vi "Update.vi"(8 "error in (no error)":errorcluster, 10 "Message in":refnum<class "UpdateMessage.lvclass">, 11 "StageSPIM in":refnum<class "StageSPIM.lvclass">) -> (0 "error out":errorcluster, 3 "StageSPIM out":refnum<class "StageSPIM.lvclass">)   [LabVIEW 2012, in "StageSPIM.lvclass"]
doc: "The update method processes the command 'update'. \n\nThe command 'update' is used for receiving new values to be set to the private data of the class. This could be seen as a public set method for setting new parameters to the private class data."
uses:
  StageSPIM.lvclass
  <vilib>/Distrio/Murmex/Murmex/Murmex.lvclass
  <vilib>/Distrio/Murmex/UpdateMessage/UpdateMessage.lvclass
panel:
  # "This method is called when the UPDATE\ntrigger is sent. \n\nOverride this method when your component needs to\nrespond to this trigger. \n\nCall parent for proper implementation"
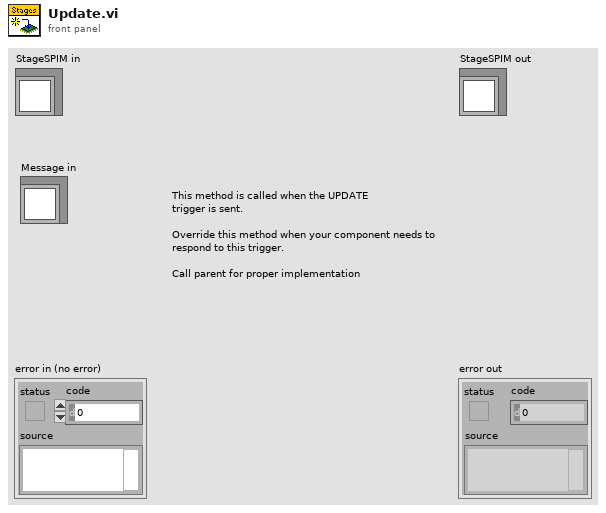
[diagram p1: front panel]
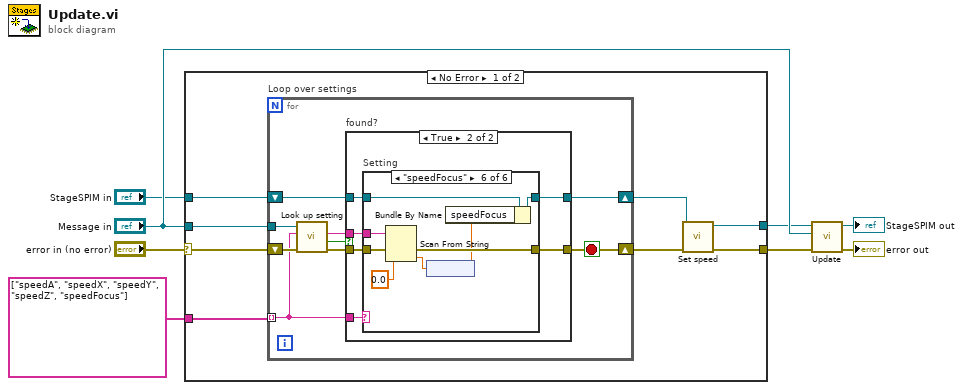
[diagram p0: block diagram]
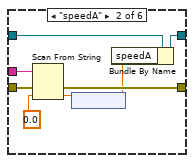
[diagram p4: hidden frame]
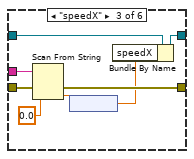
[diagram p5: hidden frame]
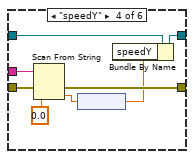
[diagram p6: hidden frame]
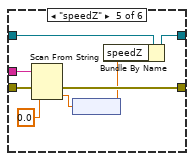
[diagram p7: hidden frame]
diagram:
  n1 = case shown="No Error" "error in (no error)" {
    selector: "error in (no error)" -> [w16 w76]
    tunnel: [w11 w76] -> w5
    tunnel: string[] ["speedA", "speedX", "speedY", "speedZ", "speedFocus"] ("key chains") -> [w15 _]
    tunnel: "Message in" -> [w14 _]
    tunnel: "StageSPIM in" -> [w13 w77]
    tunnel: [w9 w77] -> w1
    frame No Error {
      n2 = for "Loop over settings" {
        shift-right: [w17] -> w12
        shift-left: w16 -> [w25]
        tunnel: w15 -> [w19] mode=indexing
        tunnel: w14 -> [w24]
        shift-right: [w18] -> w10
        shift-left: w13 -> [w22]
        stop <- w17 stop-if-true
        n3 = call <vilib>:"Look up setting.vi"("error in (no error)"=w25, "tag name"=w19, "UpdateMessage in"=w24) -> ("error out"=w20:errorcluster, "found?"=w23:bool, "value"=w21:string)  [unwired: 5 in, 1 out]
        n4 = case "found?" shown="True" w23 {
          tunnel: w22 -> [w27 w31]
          tunnel: w21 -> [_ w32]
          tunnel: w20 -> [w26 w30]
          tunnel: w19 -> [_ w33]
          tunnel: [w27 w29] -> w18
          tunnel: [w26 w28] -> w17
          frame False {
          }
          frame True {
            n5 = case "Setting" shown="\"speedFocus\"" w33 {
              tunnel: w32 -> [_ w39 w50 w54 w63 w71]
              tunnel: w31 -> [w35 w41 w49 w58 w66 w74]
              tunnel: w30 -> [w34 w43 w51 w59 w67 w75]
              tunnel: [w35 w40 w48 w57 w65 w73] -> w29
              tunnel: [w34 w42 w47 w55 w64 w72] -> w28
              frame Default {
              }
              frame "speedA" {
                n6 = Scan From String(input string=w39, error in=w43, default 1=0.0 ("Settings_cluster.Power")) -> (error out=w42:errorcluster, output 1=w38:dbl)  [unwired: 2 in, 2 out]
                n7 = node(w38) -> (w37:dbl[unit])
                n8 = Bundle By Name(cluster=w41, "speedA"=w37) -> (w40:refnum<class "StageSPIM.lvclass">)
              }
              frame "speedX" {
                n9 = Scan From String(input string=w50, error in=w51, default 1=0.0 ("Settings_cluster.Power")) -> (error out=w47:errorcluster, output 1=w46:dbl)  [unwired: 2 in, 2 out]
                n10 = node(w46) -> (w45:dbl[unit])
                n11 = Bundle By Name(cluster=w49, "speedX"=w45) -> (w48:refnum<class "StageSPIM.lvclass">)
              }
              frame "speedY" {
                n12 = Scan From String(input string=w54, error in=w59, default 1=0.0 ("Settings_cluster.Power")) -> (error out=w55:errorcluster, output 1=w53:dbl)  [unwired: 2 in, 2 out]
                n13 = node(w53) -> (w52:dbl[unit])
                n14 = Bundle By Name(cluster=w58, "speedY"=w52) -> (w57:refnum<class "StageSPIM.lvclass">)
              }
              frame "speedZ" {
                n15 = Scan From String(input string=w63, error in=w67, default 1=0.0 ("Settings_cluster.Power")) -> (error out=w64:errorcluster, output 1=w62:dbl)  [unwired: 2 in, 2 out]
                n16 = node(w62) -> (w61:dbl[unit])
                n17 = Bundle By Name(cluster=w66, "speedZ"=w61) -> (w65:refnum<class "StageSPIM.lvclass">)
              }
              frame "speedFocus" {
                n18 = Scan From String(input string=w71, error in=w75, default 1=0.0 ("Settings_cluster.Power")) -> (error out=w72:errorcluster, output 1=w70:dbl)  [unwired: 2 in, 2 out]
                n19 = node(w70) -> (w69:dbl[unit])
                n20 = Bundle By Name(cluster=w74, "speedFocus"=w69) -> (w73:refnum<class "StageSPIM.lvclass">)
              }
            }
          }
        }
      }
      n21 = call-dynamic "Set speed.vi"("error in (no error)"=w12, "StageSPIM in"=w10) -> ("error out"=w11:errorcluster, "StageSPIM out"=w9:refnum<class "StageSPIM.lvclass">)  [unwired: 8 in]
    }
    frame Error {
    }
  }
  n22 = call-parent "Update.vi"("error in (no error)"=w5, "Message in"="Message in", "Murmex in"=w1) -> ("error out"=→"error out":errorcluster, "Murmex out"=→"StageSPIM out":refnum<class "StageSPIM.lvclass">)  [unwired: 7 in]
